vi "SwapInstanceVIUnusedName2 51.vi"(6 "Bindata & descr in":T1, 7 "type":i64, 8 "error in (no error)":errorcluster, 9 "dims":u8=3 min=1 max=3, 11 "kwarg_name":string="testarg") -> (0 "error out":errorcluster, 1 "Array 3D":i64[][][](array[numeric]), 2 "Array 2D":i64[][](array[numeric]), 3 "Array 1D":i64[](array[numeric]), 4 "Bindata & descr out":T1, 5 "bindata":u8[](array[numeric]))   [LabVIEW 2018]
uses:
  Bindata&description.ctl
  Bindata description.ctl
  dc891200-ae43-4959-9315-4ed45b65dfd4.vi
  aedcc82e-2f0f-409f-a6b5-6685829a8eba.vi
  25d9e3c8-e1fb-4344-bf52-a7f0db29612a.vi
  48be39ca-10c4-4e3d-a0a4-706ef46d60d0.vi
  aedcc82e-2f0f-409f-a6b5-6685829a8eba.vi/24803c09-0dc3-4d80-8def-9db2362a368b.vi
  25d9e3c8-e1fb-4344-bf52-a7f0db29612a.vi/11d7ee54-8186-4b11-b437-3020d53eebc6.vi
  48be39ca-10c4-4e3d-a0a4-706ef46d60d0.vi/18db1641-e6f4-4638-9208-b9d7c9739f3b.vi
  aedcc82e-2f0f-409f-a6b5-6685829a8eba.vi/24803c09-0dc3-4d80-8def-9db2362a368b.vi/3ce3ef94-b667-4f42-aad9-f71ff03cd2ef.vi
  25d9e3c8-e1fb-4344-bf52-a7f0db29612a.vi/11d7ee54-8186-4b11-b437-3020d53eebc6.vi/308ec7cb-3427-4de6-875e-52f82d6271b8.vi
  48be39ca-10c4-4e3d-a0a4-706ef46d60d0.vi/18db1641-e6f4-4638-9208-b9d7c9739f3b.vi/a5e36463-8e47-4ffc-8a57-a656d3d87a66.vi
  aedcc82e-2f0f-409f-a6b5-6685829a8eba.vi/24803c09-0dc3-4d80-8def-9db2362a368b.vi/3ce3ef94-b667-4f42-aad9-f71ff03cd2ef.vi/9f2a3b29-27df-466f-9cb2-319570cc30b8.vi
  25d9e3c8-e1fb-4344-bf52-a7f0db29612a.vi/11d7ee54-8186-4b11-b437-3020d53eebc6.vi/308ec7cb-3427-4de6-875e-52f82d6271b8.vi/3364222f-7828-43b1-8c2a-fd3c42e90a6d.vi
  48be39ca-10c4-4e3d-a0a4-706ef46d60d0.vi/18db1641-e6f4-4638-9208-b9d7c9739f3b.vi/a5e36463-8e47-4ffc-8a57-a656d3d87a66.vi/e2ae0c10-b5af-4a99-82e9-a55586654c03.vi
  check ID validity.vi
  LV-Julia_ZMQ-Roundtrip_lib.lvlib
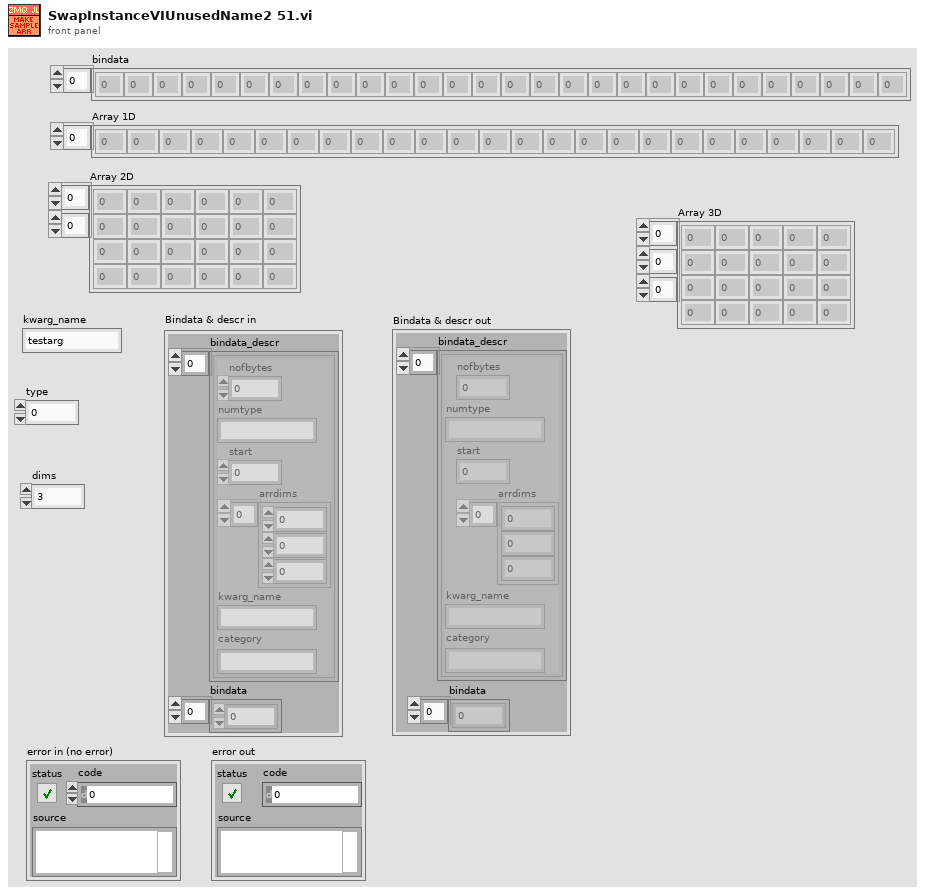
[diagram p1: front panel]
types:
  T1 = typedef "Bindata&description.ctl" = cluster{"bindata_descr":T2[], "bindata":u8[]}
  T2 = typedef "LV-Julia_ZMQ-Roundtrip_lib.lvlib/Bindata description.ctl" = cluster{"nofbytes":i32, "numtype":string, "start":i32, "arrdims":i32[], "kwarg_name":string, "category":string}
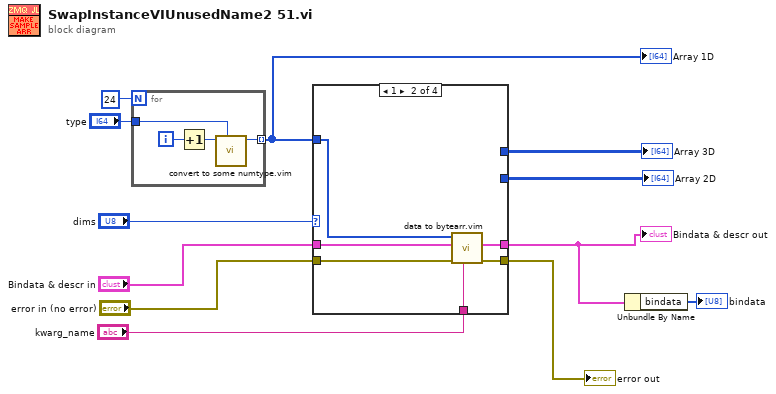
[diagram p0: block diagram]
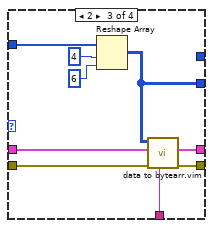
[diagram p3: hidden frame]
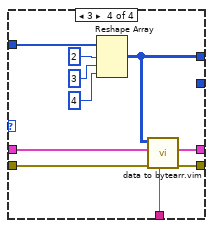
[diagram p4: hidden frame]
diagram:
  n1 = for {
    N: 24 -> [_]
    tunnel: [w14] -> w11 mode=indexing
    tunnel: "type" -> [w13]
    i -> [w16]
    n2 = Increment(x=w16) -> (x+1=w15:i32)
    n3 = call "convert to some numtype.vim"("type"=w13, "Numeric in"=w15) -> ("Numeric out"=w14:i64)  [unwired: 9 in]
  }
  "Array 1D" <- w11
  n4 = case shown="1" "dims" {
    tunnel: [_ _ _ w42] -> w12
    tunnel: w11 -> [_ w23 w30 w38]
    tunnel: "kwarg_name" -> [_ w22 w29 w37]
    tunnel: "error in (no error)" -> [w17 w21 w28 w36]
    tunnel: [w17 w20 w27 w35] -> w5
    tunnel: [_ w19 w26 w34] -> w2
    tunnel: [_ _ w25 _] -> w4
    tunnel: "Bindata & descr in" -> [_ w18 w24 w33]
    frame 0, Default {
    }
    frame 1 {
      n5 = call "data to bytearr.vim"("kwarg_name"=w22, "error in (no error)"=w21, "Bindata & descr in"=w18, "data in"=w23) -> ("error out"=w20:errorcluster, "Bindata & descr out"=w19:T1)  [unwired: 5 in, 1 out]
    }
    frame 2 {
      n6 = Reshape Array(w30, 4 ("dimension size"), 6 ("dimension size")) -> (w25:i64[][])
      n7 = call "data to bytearr.vim"("kwarg_name"=w29, "error in (no error)"=w28, "Bindata & descr in"=w24, "data in"=w25) -> ("error out"=w27:errorcluster, "Bindata & descr out"=w26:T1)  [unwired: 5 in, 1 out]
    }
    frame 3 {
      n8 = Reshape Array(w38, 2 ("dimension size"), 3 ("dimension size"), 4 ("dimension size")) -> (w42:i64[][][])
      n9 = call "data to bytearr.vim"("kwarg_name"=w37, "error in (no error)"=w36, "Bindata & descr in"=w33, "data in"=w42) -> ("error out"=w35:errorcluster, "Bindata & descr out"=w34:T1)  [unwired: 5 in, 1 out]
    }
  }
  "Array 3D" <- w12
  "Bindata & descr out" <- w2
  "error out" <- w5
  "Array 2D" <- w4
  n10 = Unbundle By Name(w2) -> ("bindata"=→"bindata":u8[])
